vi "#Counter.vi"(8 "error in":errorcluster, 11 "Enum":enum16{"Count Time", "Pause Time", "Reset Time"}(ring)) -> (0 "error out":errorcluster, 3 "Elapsed Time":dbl)   [LabVIEW 2023]
panel:
  out "Pause Time":dbl
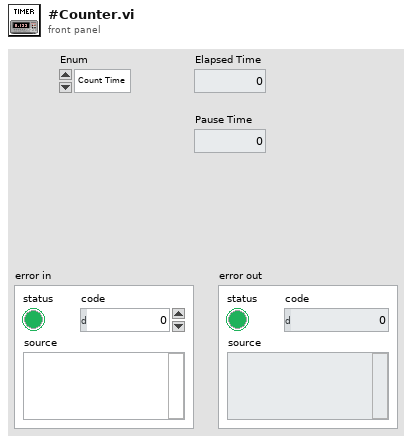
[diagram p1: front panel]
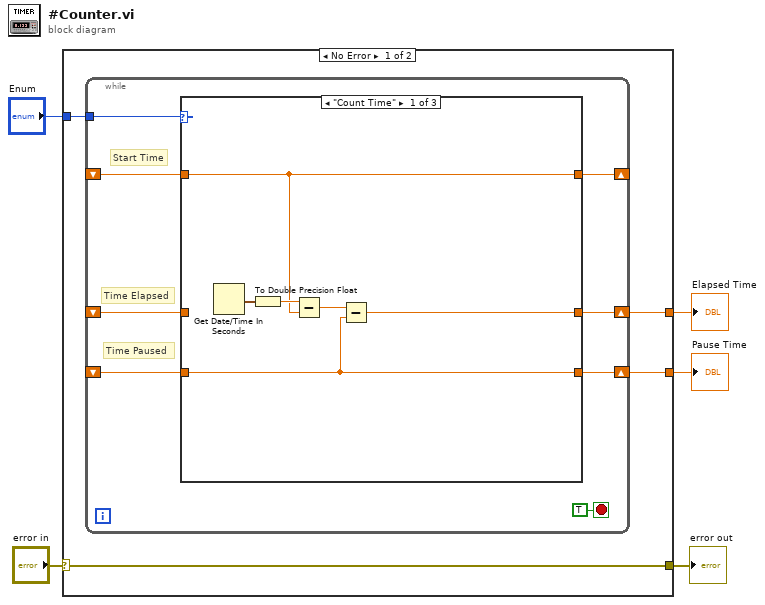
[diagram p0: block diagram]
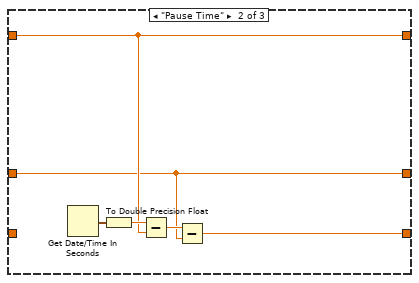
[diagram p2: hidden frame]
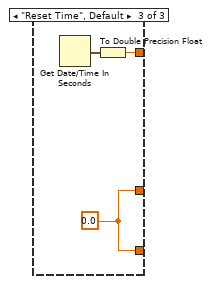
[diagram p3: hidden frame]
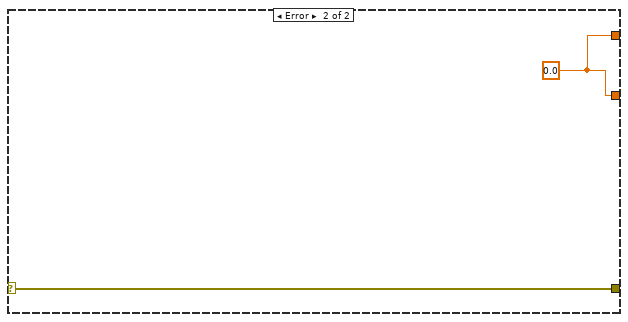
[diagram p4: hidden frame]
diagram:
  n1 = case shown="No Error" "error in" {
    selector: "error in" -> [w6 w34]
    tunnel: "Enum" -> [w9 _]
    tunnel: [w8 w33] -> w3
    tunnel: [w7 w33] -> w2
    tunnel: [w6 w34] -> w1
    frame No Error {
      n2 = while {
        tunnel: w9 -> [w17]
        shift-right: [w14] -> w7
        shift-left: _ -> [w13]
        shift-right: [w15] -> w8
        shift-left: _ -> [w12]
        shift-right: [w11] -> _
        shift-left: _ -> [w10]
        stop <- TRUE stop-if-true
        # "Start Time"
        # "Time Paused"
        # "Time Elapsed"
        n3 = case shown="\"Count Time\"" w17 {
          tunnel: [w19 w24 w32] -> w14
          tunnel: [w18 w25 w32] -> w15
          tunnel: w13 -> [_ w24 _]
          tunnel: w12 -> [w18 _ _]
          tunnel: [w20 w27 w30] -> w11
          tunnel: w10 -> [w20 w27 _]
          frame "Count Time" {
            n4 = Get Date/Time In Seconds() -> (seconds since 1Jan1904=w23:timestamp)
            n5 = To Double Precision Float(number=w23) -> (double precision float=w22:dbl)
            n6 = Subtract(x=w22, y=w20) -> (x-y=w21:dbl)
            n7 = Subtract(x=w21, y=w18) -> (x-y=w19:dbl)
          }
          frame "Pause Time" {
            n8 = Get Date/Time In Seconds() -> (seconds since 1Jan1904=w29:timestamp)
            n9 = To Double Precision Float(number=w29) -> (double precision float=w28:dbl)
            n10 = Subtract(x=w28, y=w27) -> (x-y=w26:dbl)
            n11 = Subtract(x=w26, y=w24) -> (x-y=w25:dbl)
          }
          frame "Reset Time", Default {
            w32 = 0.0
            n12 = Get Date/Time In Seconds() -> (seconds since 1Jan1904=w31:timestamp)
            n13 = To Double Precision Float(number=w31) -> (double precision float=w30:dbl)
          }
        }
      }
    }
    frame Error {
      w33 = 0.0
    }
  }
  "Elapsed Time" <- w2
  "Pause Time" <- w3
  "error out" <- w1
